vi "Verify_Stable_Voltage.vi"(8 "Error in":errorcluster) -> (0 "Error out":errorcluster, 5 "Voltage Stable":bool)   [LabVIEW 2020]
panel:
  out "Voltage out":dbl format="%0.6f"
  out "Loops":i32
  in  "Sample 2":dbl format="%#_13g"
  in  "Sample 1":dbl format="%#_13g"
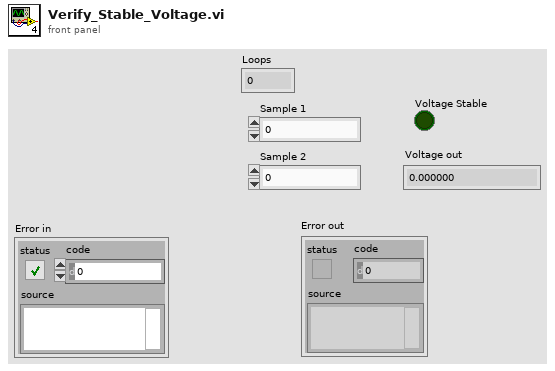
[diagram p1: front panel]
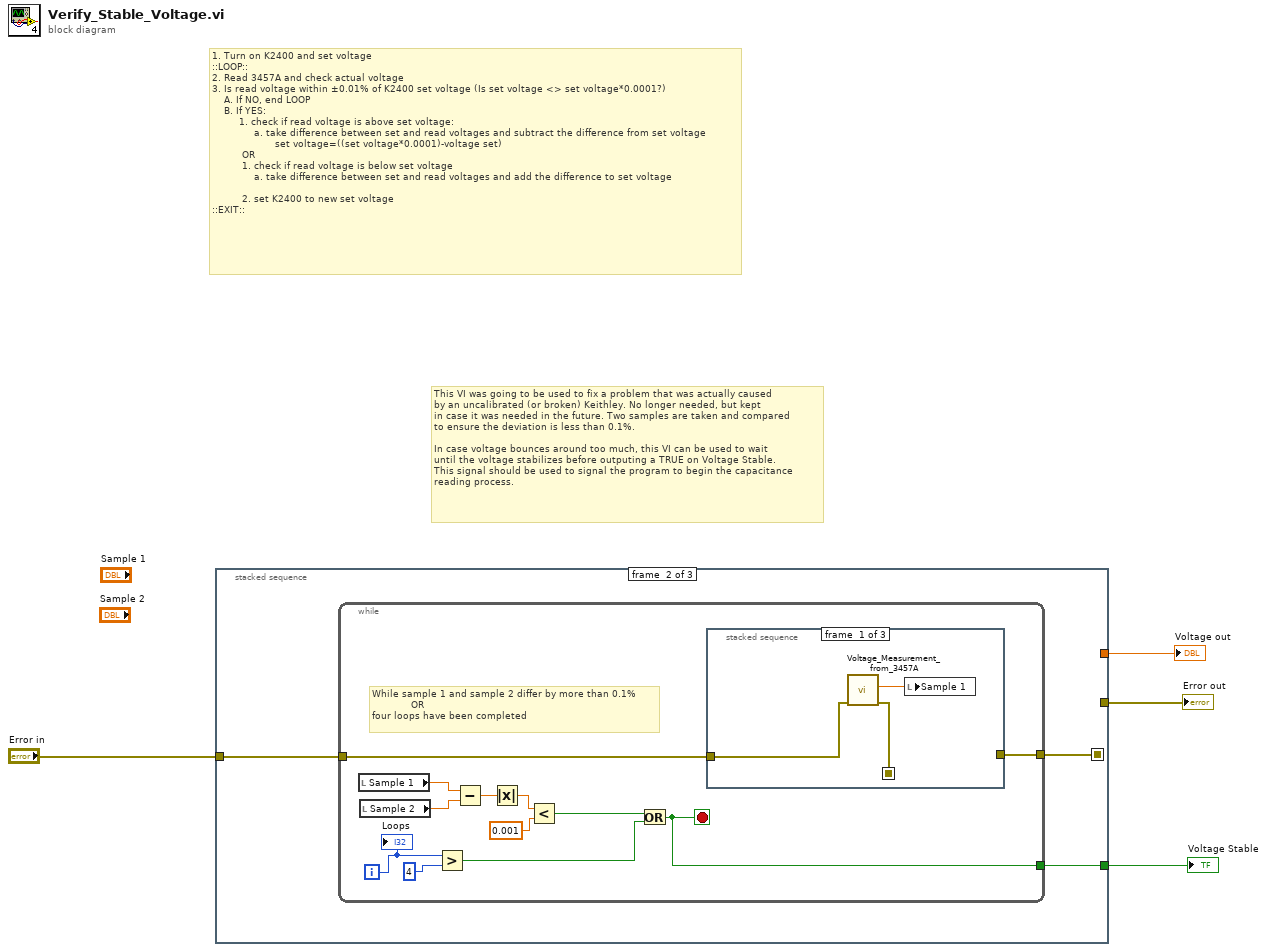
[diagram p0: block diagram]
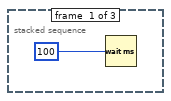
[diagram p2: hidden frame]
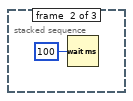
[diagram p3: hidden frame]
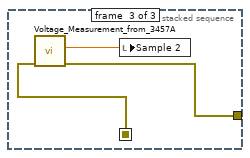
[diagram p4: hidden frame]
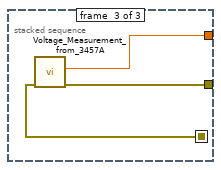
[diagram p5: hidden frame]
diagram:
  # "This VI was going to be used to fix a problem that was actually caused\nby an uncalibrated (or broken) Keithley. No longer needed, but kept\nin case it was needed in the future. Two samples are taken and compared\nto ensure the deviation is less than 0.1%.\n\nIn case voltage bounces around too much, this VI can be used to wait\nuntil the voltage stabilizes before outputing a TRUE on Voltage Stable.\nThis signal should be used to signal the program to begin the capacitance\nreading process."
  # "1. Turn on K2400 and set voltage\n::LOOP::\n2. Read 3457A and check actual voltage\n3. Is read voltage within ±0.01% of K2400 set voltage (Is set voltage <> set voltage*0.0001?)\n    A. If NO, end LOOP\n    B. If YES:\n         1. check if read voltage is above set voltage:\n              a. take difference between set and read voltages and subtract the difference from set voltage\n                     set voltage=((set voltage*0.0001)-voltage set)\n          OR\n          1. check if read voltage is below set voltage\n              a. take difference between set and read voltages and add the difference to set voltage\n\n          2. set K2400 to new set voltage\n::EXIT::"
  n1 = stacked-sequence {
    seq-local: [_ w6 _] -> [_ _ w29]
    tunnel: "Error in" -> [_ w7 _]
    tunnel: [_ _ w30] -> w4
    tunnel: [_ w8 _] -> w3
    tunnel: [_ _ w28] -> w1
    frame #0 {
      n2 = Wait (ms)(milliseconds to wait=u32 100) -> ()  [unwired: 1 out]
    }
    frame #1 {
      n3 = while {
        tunnel: [w11] -> w8
        tunnel: w7 -> [w10]
        tunnel: [w9] -> w6
        i -> [w18]
        stop <- w11 stop-if-true
        # "While sample 1 and sample 2 differ by more than 0.1%\n             OR\nfour loops have been completed"
        n4 = local read "Sample 1"() -> (w17:dbl)
        n5 = local read "Sample 2"() -> (w16:dbl)
        n6 = Greater?(x=w18, y=4) -> (0:w20:bool)
        n7 = Subtract(x=w17, y=w16) -> (x-y=w15:dbl)
        n8 = Absolute Value(x=w15) -> (abs(x)=w13:dbl)
        n9 = Less?(x=w13, y=0.001 ("upper limit")) -> (x < y?=w12:bool)
        n10 = Or(x=w12, y=w20) -> (x .or. y?=w11:bool)
        n11 = stacked-sequence {
          seq-local: [w22 _ _] -> [_ _ w27]
          tunnel: w10 -> [w21 _ _]
          tunnel: [_ _ w25] -> w9
          frame #0 {
            n12 = call "Voltage_Measurement_from_3457A.vi"("error in"=w21) -> ("error out"=w22:errorcluster, "mean"=w23:dbl)  [unwired: 9 in]
            n13 = local write "Sample 1"(w23) -> ()
          }
          frame #1 {
            n14 = Wait (ms)(milliseconds to wait=u32 100) -> ()  [unwired: 1 out]
          }
          frame #2 {
            n15 = call "Voltage_Measurement_from_3457A.vi"("error in"=w27) -> ("error out"=w25:errorcluster, "mean"=w26:dbl)  [unwired: 9 in]
            n16 = local write "Sample 2"(w26) -> ()
          }
        }
        "Loops" <- w18
      }
    }
    frame #2 {
      n17 = call "Voltage_Measurement_from_3457A.vi"("error in"=w29) -> ("error out"=w30:errorcluster, "mean"=w28:dbl)  [unwired: 9 in]
    }
  }
  "Error out" <- w4
  "Voltage Stable" <- w3
  "Voltage out" <- w1
